vi "DIO Set.vi"(7 "Box ID":u8, 8 "error in (no error)":errorcluster, 9 "DIO Enable":bool[](array[boolean]), 10 "DIO Direction":bool[](array[boolean]), 11 "ENET in":refnum<class "ENET_BS120x.lvclass">) -> (0 "error out":errorcluster, 3 "ENET out":refnum<class "ENET_BS120x.lvclass">)   [LabVIEW 2021, in "BS120x Driver.lvlib" / "ENET_BS120x.lvclass"]
uses:
  ENET_BS120x.lvclass
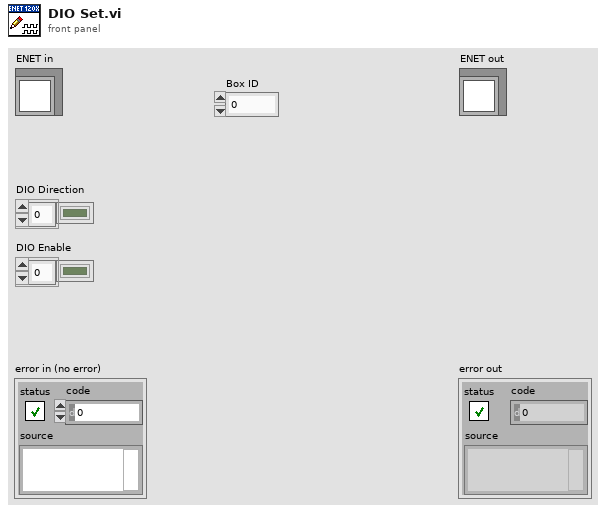
[diagram p1: front panel]
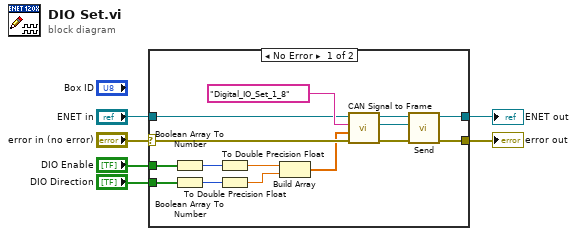
[diagram p0: block diagram]
diagram:
  n1 = case shown="No Error" "error in (no error)" {
    selector: "error in (no error)" -> [w16 w22]
    tunnel: [w17 w22] -> w6
    tunnel: "DIO Direction" -> [w11 _]
    tunnel: "DIO Enable" -> [w10 _]
    tunnel: "ENET in" -> [w8 w23]
    tunnel: [w7 w23] -> w3
    frame No Error {
      n2 = Boolean Array To Number(Boolean array=w10) -> (number=w13:u32)
      n3 = Boolean Array To Number(Boolean array=w11) -> (number=w12:u32)
      n4 = To Double Precision Float(number=w13) -> (double precision float=w14:dbl)
      n5 = To Double Precision Float(number=w12) -> (double precision float=w15:dbl)
      n6 = Build Array(w14, w15) -> (w9:dbl[])
      n7 = call "CAN Signal to Frame.vi"("error in (no error)"=w16, "Data Array"=w9, "Frame"="Digital_IO_Set_1_8", "ENET in"=w8) -> ("error out"=w18:errorcluster, "Data"=w19:refnum<class "Data.lvclass">, "ENET out"=w20:refnum<class "ENET_BS120x.lvclass">)  [unwired: 5 in]
      n8 = call "Send.vi"("error in (no error)"=w18, "Data"=w19, "ENET in"=w20) -> ("error out"=w17:errorcluster, "ENET out"=w7:refnum<class "ENET_BS120x.lvclass">)  [unwired: 7 in]
    }
    frame Error {
    }
  }
  "error out" <- w6
  "ENET out" <- w3
